vi "fpga_status.vi"(8 "error in (no error)":errorcluster, 11 "5785_2_x_1600MHz in":refnum<class "5785_2_x_1600MHz.lvclass">) -> (0 "error out":errorcluster, 2 "pulse TX status":T1, 3 "5785_2_x_1600MHz out":refnum<class "5785_2_x_1600MHz.lvclass">)   [LabVIEW 2021, in "5785_2_x_1600MHz.lvclass"]
uses:
  5785_2_x_1600MHz.lvclass
  5785_2_x_1600MHz.lvclass/5785_2_x_1600MHz.ctl
  <vilib>/Utility/error.llb/Error Cluster From Error Code.vi
  <vilib>/rvi/errors/niLvFpgaAdjustHostInterfaceError.vi
  <vilib>/rvi/interface/nirviReadWriteControl/nirviReadWriteControl.xnode
  NiFpgaLv.dll
  <vilib>/rvi/interface/Simulation/niFpgaSimulationCallBeginRW.vi
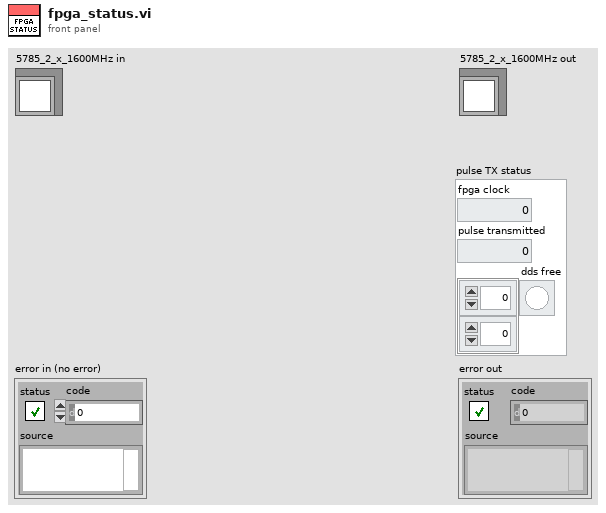
[diagram p1: front panel]
types:
  T1 = cluster{"fpga clock":dbl, "pulse transmitted":u32, "dds free":bool[][]}
  T2 = cluster{"fpga clock":u64, "pulse transmitted":u32, "dds free":bool[]}
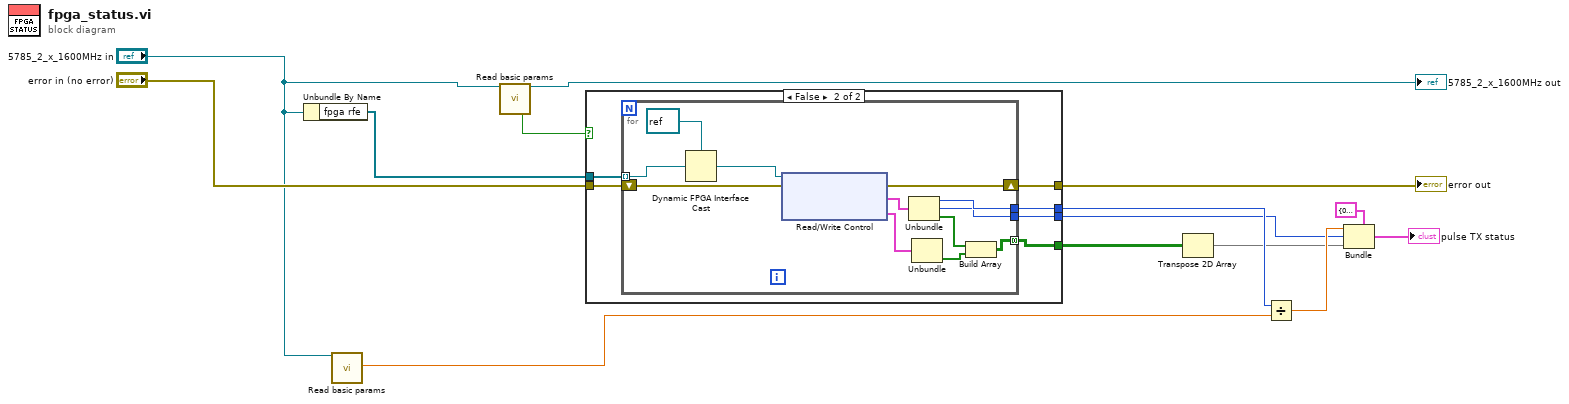
[diagram p0: block diagram]
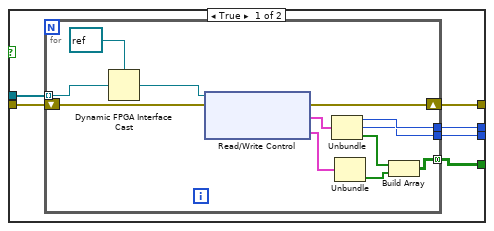
[diagram p2: hidden frame]
diagram:
  n1 = Unbundle By Name("5785_2_x_1600MHz in") -> ("fpga rfe"=w14:refnum<k20>[])
  n2 = call-dynamic "Read basic params.vi"("device_type in"="5785_2_x_1600MHz in") -> ("Fs  FPGA"=w10:dbl)  [unwired: 12 in, 6 out]
  n3 = call-dynamic "Read basic params.vi"("device_type in"="5785_2_x_1600MHz in") -> ("use arb files"=w1:bool, "device_type out"=→"5785_2_x_1600MHz out":refnum<class "5785_2_x_1600MHz.lvclass">)  [unwired: 12 in, 5 out]
  n4 = case shown="False" w1 {
    tunnel: w14 -> [w20 w38]
    tunnel: "error in (no error)" -> [w19 w37]
    tunnel: [w18 w36] -> w12
    tunnel: [w17 w35] -> w11
    tunnel: [w16 w34] -> w6
    tunnel: [w15 w33] -> w5
    frame True {
      n5 = for {
        tunnel: w20 -> [w23] mode=indexing
        tunnel: [w29] -> w17
        tunnel: [w28] -> w16
        shift-right: [w31] -> w18
        shift-left: w19 -> [w32]
        tunnel: [w26] -> w15 mode=concatenating
        n6 = Dynamic FPGA Interface Cast(Session In=refnum<k20> refnum ("Type"), Type=w23) -> (Session Out=w22:refnum<k20>)
        n7 = xnode "Read/Write Control"("FPGA VI Reference In"=w22, "error in"=w32) -> ("error out"=w31:errorcluster, "pulse TX status"=w30:T2, "pulse TX status 2"=w25:T2)  [unwired: 1 out]
        n8 = Unbundle(w30) -> ("fpga clock"=w29:u64, "pulse transmitted"=w28:u32, "dds free"=w27:bool[])
        n9 = Unbundle(w25) -> ("dds free"=w24:bool[])  [unwired: 2 out]
        n10 = Build Array(w27, w24) -> (w26:bool[][])
      }
    }
    frame False {
      n11 = for {
        tunnel: w38 -> [w41] mode=indexing
        tunnel: [w47] -> w35
        tunnel: [w46] -> w34
        shift-right: [w49] -> w36
        shift-left: w37 -> [w50]
        tunnel: [w44] -> w33 mode=concatenating
        n12 = Dynamic FPGA Interface Cast(Session In=refnum<k20> refnum ("Type"), Type=w41) -> (Session Out=w40:refnum<k20>)
        n13 = xnode "Read/Write Control"("FPGA VI Reference In"=w40, "error in"=w50) -> ("error out"=w49:errorcluster, "pulse TX status"=w48:T2, "pulse TX status 2"=w43:T2)  [unwired: 1 out]
        n14 = Unbundle(w48) -> ("fpga clock"=w47:u64, "pulse transmitted"=w46:u32, "dds free"=w45:bool[])
        n15 = Unbundle(w43) -> ("dds free"=w42:bool[])  [unwired: 2 out]
        n16 = Build Array(w45, w42) -> (w44:bool[][])
      }
    }
  }
  "error out" <- w12
  n17 = Transpose 2D Array(2D array=w5) -> (transposed array=w4:bool[][])
  n18 = Divide(x=w11, y=w10) -> (x/y=w7:dbl)
  n19 = Bundle(cluster=T1 {"fpga clock"=0.0, "pulse transmitted"=0, "dds free"=[[FALSE, FALSE, FALSE, FALSE, FALSE, FALSE, FALSE, FALSE, FALSE, FALSE, FALSE, FALSE, FALSE, FALSE, FALSE, FALSE]]} ("pulse TX status"), "fpga clock"=w7, "pulse transmitted"=w6, "dds free"=w4) -> (→"pulse TX status":T1)
